vi "Handle Error.vi"(8 "error in (no error)":errorcluster, 11 "MainUI Panel in":refnum<class "MainUI Panel.lvclass">) -> (0 "error out":errorcluster, 2 "stop actor?":bool=TRUE, 3 "MainUI Panel out":refnum<class "MainUI Panel.lvclass">)   [LabVIEW 2019, in "MainUI.lvlib" / "MainUI Panel.lvlib" / "MainUI Panel.lvclass"]
doc: "(<B>Filename</B>: Actor Framework.lvlib:Actor.lvclass:Handle Error.vi)\n\nDefines how the actor handles an error that occurred while processing a message. By default, this method does nothing except stop the actor."
uses:
  MainUI Panel.lvclass
  ModuleAbstract/ModuleAbstract.lvclass
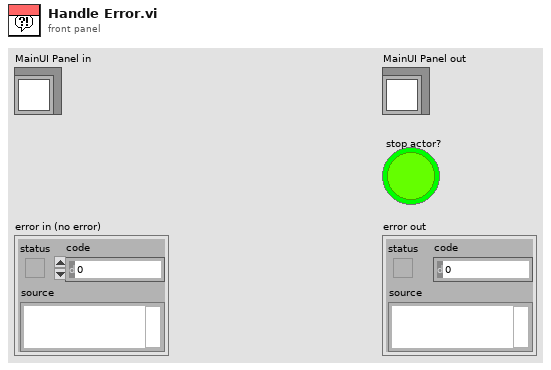
[diagram p1: front panel]
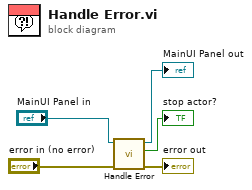
[diagram p0: block diagram]
diagram:
  n1 = call-parent "Handle Error.vi"("error in (no error)"="error in (no error)", "ModuleAbstract in"="MainUI Panel in") -> ("error out"=→"error out":errorcluster, "stop actor?"=→"stop actor?":bool, "ModuleAbstract out"=→"MainUI Panel out":refnum<class "MainUI Panel.lvclass">)  [unwired: 7 in]
